vi "Day6_Logging.vi"() -> ()   [LabVIEW 2025]
uses:
  <vilib>/Platform/TimedLoop/XDataNode/timing_clust.ctl
  <vilib>/Platform/TimedLoop/XDataNode/nitl_modes.ctl
  <vilib>/Platform/TimedLoop/XDataNode/wakeup.ctl
  <vilib>/Utility/error.llb/Trim Whitespace One-Sided.vi
  <vilib>/Instr/_visa.llb/VISA Configure Serial Port (Instr).vi
  <vilib>/Utility/file.llb/Write Delimited Spreadsheet (DBL).vi
  <vilib>/platform/TimedLoop/XDataNode/XDataNode.xnode
  <vilib>/Platform/TimedLoop/XDataNode/XDNodeRunTimeDep.lvlib
  <vilib>/ptbypt/NI_PtbyPt.lvlib
panel:
  in  "Log File Path":path
  out "Touch FAIL":bool
  out "Touch PASS":bool
  in  "Touch Lo Limit":dbl
  in  "Touch Hi Limit":dbl
  out "Max":dbl
  out "Min":dbl
  out "Mean":dbl
  out "Std Dev":dbl
  out "mean":dbl format="%0.2f"
  out "ADC (mv)":dbl
  out "Touch Pin":dbl
  out "Hall Sensor":dbl
  out "Timestamp":dbl
  in  "stop":bool
  # "Day 4: Statistics engine using a custom SubVI. Collects last 20 Touch Pin readings and computes live stats"
  # "Mean PtByPt: continuous running average since session start"
  # "Stats SubVI outputs: computed from a rolling buffer of the last 20 Touch Pin samples."
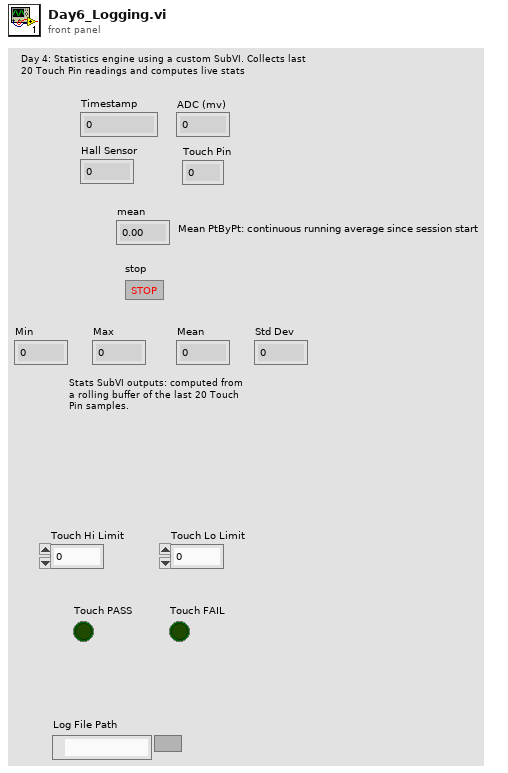
[diagram p1: front panel]
types:
  T1 = typedef "XDNodeRunTimeDep.lvlib/timing_clust.ctl" = cluster{"Expected End [f-1]":u64, "Actual End [f-1]":u64, "Finished Late? [f-1]":bool, "Expected End [i-1]":u64, "Actual End [i-1]":u64, "Finished Late? [i-1]":bool, "Expected Start [i]":u64, "Actual Start [i]":u64, "Expected Start [f]":u64, "Actual Start [f]":u64, "Source Name":string, "Structure Name":string, "Period":i64, "Deadline":i64, "Offset":i64, "Start":i64, "Priority":i32, "Timeout":i32, "Mode":T2, "Wakeup Reason":T3, "Error":errorcluster, "Source Type":string, "Secondary Source Type":string, "Global End Time":u64, "Global Start Time":u64, "Frame Duration":u64, "Iteration Duration":u64, "Assigned CPU":i32, "I/O Scan Engine Mode":u32}
  T2 = typedef "XDNodeRunTimeDep.lvlib/nitl_modes.ctl" = enum32{"No Change", "Process missed periods, maintain original phase", "Discard missed periods, maintain original phase", "Process missed periods, ignore original phase", "Discard missed periods, ignore original phase"}
  T3 = typedef "XDNodeRunTimeDep.lvlib/wakeup.ctl" = enum32{"Normal", "Aborted", "Asynchronous wakeup", "Timing source error", "Timed loop error", "Timeout"}
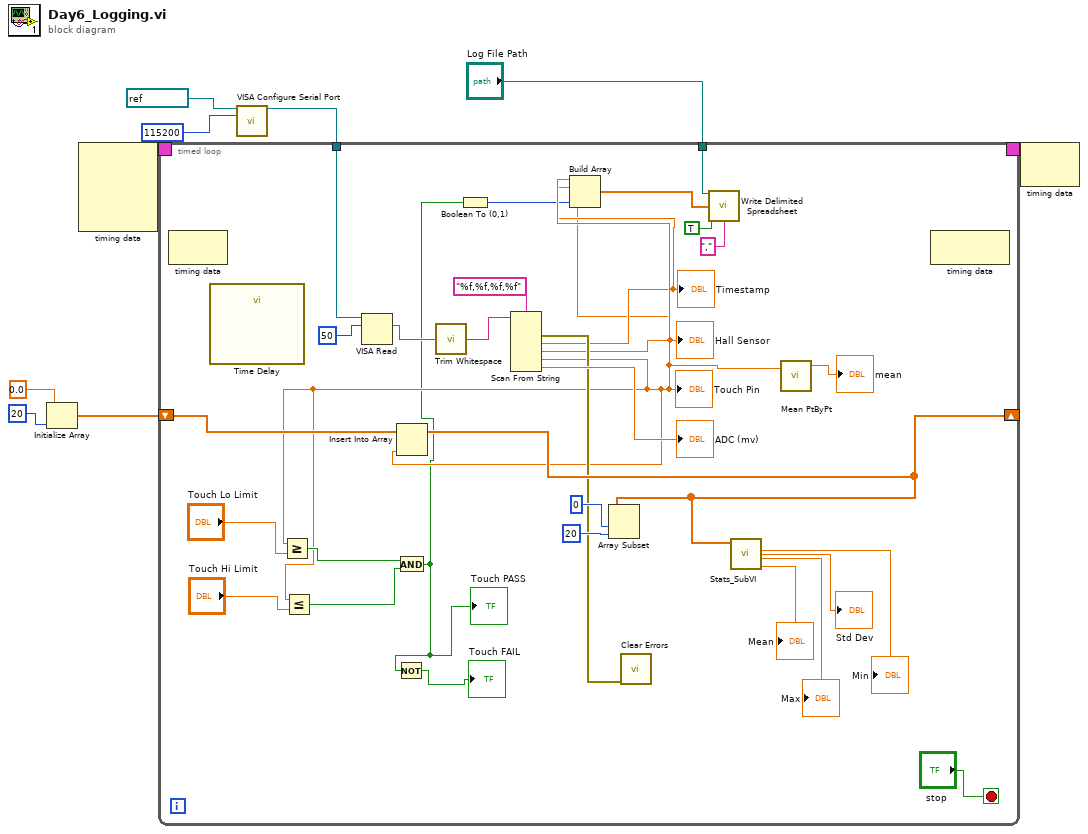
[diagram p0: block diagram]
diagram:
  n1 = Initialize Array "Initialize Array"(0.0 ("element"), 20 ("dimension size")) -> (w4:dbl[])
  n2 = node-c288() -> (w7:T1)  [unwired: 4 in]
  n3 = call-poly "VISA Configure Serial Port"("VISA resource name"=refnum<visa-resource-name> "COM4", "baud rate (9600)"=u32 115200) -> ("VISA resource name out"=w5:refnum<visa-resource-name>)  [unwired: 12 in, 1 out]
  n4 = timed-loop {
    timing: w7 -> [_]
    timing-out: [_] -> w6
    tunnel: w5 -> [w35]
    shift-right: [w29] -> _
    shift-left: w4 -> [w32]
    tunnel: "Log File Path" -> [w12]
    stop <- "stop" stop-if-true
    n5 = node-c288() -> ()  [unwired: 1 in, 1 out]
    n6 = call "Time Delay"() -> ()  [unwired: 11 in, 1 out]
    n7 = VISA Read(VISA resource name=w35, byte count=u32 50) -> (read buffer=w39:string)  [unwired: 1 in, 3 out]
    n8 = call <vilib>:"Trim Whitespace.vi"("string"=w39) -> ("trimmed string"=w38:string)  [unwired: 1 in]
    n9 = Scan From String "Scan From String"(format string="%f,%f,%f,%f", input string=w38) -> (error out=w20:errorcluster, output 1=w16:dbl, output 2=w15:dbl, output 3=w18:dbl, output 4=→"ADC (mv)":dbl)  [unwired: 6 in, 2 out]
    "Timestamp" <- w16
    "Hall Sensor" <- w15
    "Touch Pin" <- w18
    n10 = Greater Or Equal?(x=w18, y="Touch Lo Limit") -> (x >= y?=w23:bool)
    n11 = Less Or Equal?(x=w18, y="Touch Hi Limit") -> (x <= y?=w22:bool)
    n12 = Insert Into Array "Insert Into Array"(array=w32, new element=w18) -> (w29:dbl[])  [unwired: 1 in]
    n13 = And(x=w23, y=w22) -> (x .and. y?=w14:bool)
    "Touch PASS" <- w14
    n14 = Not(x=w14) -> (.not. x?=→"Touch FAIL":bool)
    n15 = Boolean To (0,1)(Boolean=w14) -> (0, 1=w13:i16)
    n16 = Build Array "Build Array"(w18, w16, w15, w13) -> (w17:dbl[])
    n17 = Array Subset "Array Subset"(array=w29, index=0, length=20) -> ()  [unwired: 1 out]
    n18 = call <vilib>:"Clear Errors.vi"("error in (no error)"=w20) -> ()  [unwired: 5 in, 2 out]
    n19 = call-poly <vilib>:"Write Delimited Spreadsheet.vi"("file path (dialog if empty)"=w12, "1D data"=w17, "append to file? (new file:F)"=TRUE, "delimiter (\\t)"="," ("delimiter (\\t)")) -> ()  [unwired: 10 in, 2 out]
    n20 = call "Stats_SubVI.vi"("Input Array"=w29) -> ("Std Dev"=→"Std Dev":dbl, "Mean"=→"Mean":dbl, "Max"=→"Max":dbl, "Min"=→"Min":dbl)
    n21 = call <vilib>:"Mean PtByPt.vi"("x"=w18) -> ("mean"=→"mean":dbl)  [unwired: 3 in, 1 out]
    n22 = node-c288() -> ()  [unwired: 1 in, 1 out]
  }
  n23 = node-c288(w6) -> ()  [unwired: 1 out]
